vi "Show the Schemas.vi"(8 "error in (no error)":errorcluster, 11 "Import Export SQL in":refnum<class "Import Export SQL.lvclass">) -> (0 "error out":errorcluster, 3 "Import Export SQL out":refnum<class "Import Export SQL.lvclass">)   [LabVIEW 2023, in "Data Analysis.lvlib" / "Import Export SQL.lvlib" / "Import Export SQL.lvclass"]
uses:
  Import Export SQL.lvclass
  Import Export SQL.lvclass/Import Export SQL.ctl
  HardwareAbstractionLayer_LVOOP/Database/Database.lvclass
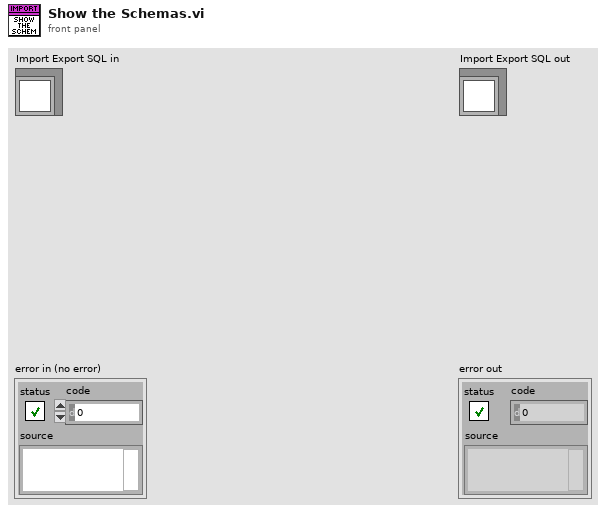
[diagram p1: front panel]
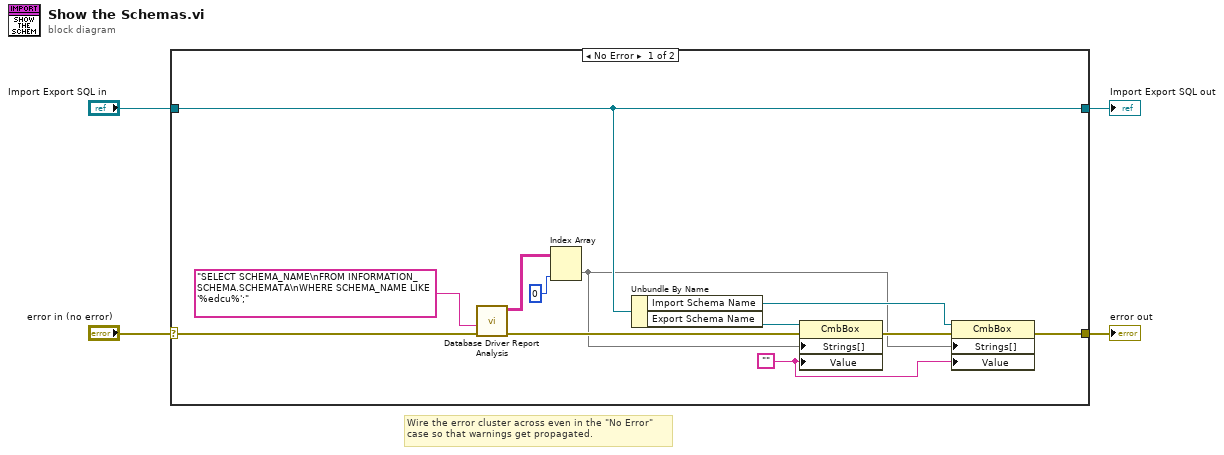
[diagram p0: block diagram]
diagram:
  # "Wire the error cluster across even in the \"No Error\"\ncase so that warnings get propagated."
  n1 = case shown="No Error" "error in (no error)" {
    selector: "error in (no error)" -> [w16 w18]
    tunnel: [w7 w18] -> w3
    tunnel: [w12 w17] -> w1
    tunnel: "Import Export SQL in" -> [w12 w17]
    frame No Error {
      w5 = ""
      n2 = call "Database Driver Report Analysis.vi"("error in"=w16, "SQL query"="SELECT SCHEMA_NAME\nFROM INFORMATION_SCHEMA.SCHEMATA\nWHERE SCHEMA_NAME LIKE '%edcu%';") -> ("error out"=w10:errorcluster, "data"=w14:string[][])  [unwired: 6 in, 2 out]
      n3 = Index Array(array=w14, index (col)=0 ("disabled index (col)")) -> (element=w6:string[])  [unwired: 1 in]
      n4 = Unbundle By Name(w12) -> ("Import Schema Name"=w9:refnum<vi>, "Export Schema Name"=w11:refnum<vi>)
      n5 = property class="CmbBox"(reference=w11, error in=w10, "Strings[]"=w6, "Value"=w5) -> (error out=w8:errorcluster)  [unwired: 1 out]
      n6 = property class="CmbBox"(reference=w9, error in=w8, "Strings[]"=w6, "Value"=w5) -> (error out=w7:errorcluster)  [unwired: 1 out]
    }
    frame Error {
    }
  }
  "error out" <- w3
  "Import Export SQL out" <- w1
